vi "AddCustomError.vi"(1 "error in (no error)":errorcluster, 2 "source":string, 3 "code":i32, 4 "Error?":bool) -> (0 "error in (no error) 2":errorcluster)   [LabVIEW 2013]
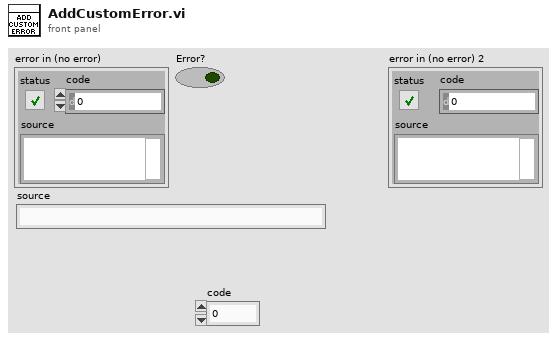
[diagram p1: front panel]
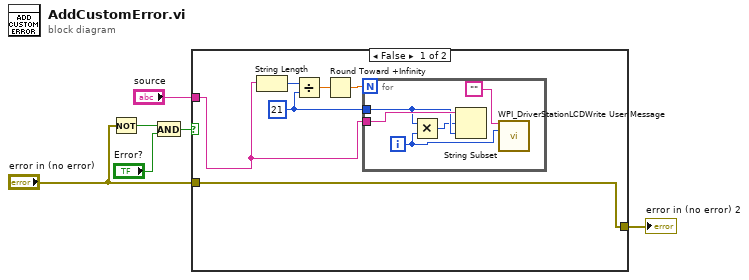
[diagram p0: block diagram]
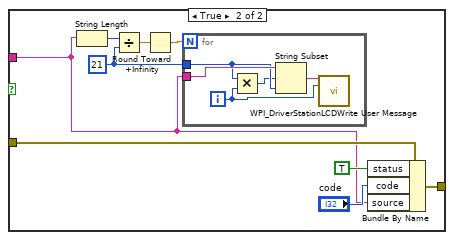
[diagram p2: hidden frame]
diagram:
  n1 = Not(x="error in (no error)") -> (.not. x?=w5:bool)
  n2 = And(x=w5, y="Error?") -> (x .and. y?=w6:bool)
  n3 = case shown="False" w6 {
    tunnel: "error in (no error)" -> [w12 w26]
    tunnel: [w12 w24] -> w2
    tunnel: "source" -> [w7 w18]
    frame False {
      w11 = 21 ("y")
      n4 = String Length(string=w7) -> (length=w8:i32)
      n5 = Divide(x=w8, y=w11) -> (x/y=w9:dbl)
      n6 = Round Toward +Infinity(x=w9) -> (ceil(x): smallest int >= x=w10:dbl)
      n7 = for {
        N: w10 -> [_]
        tunnel: w7 -> [w17]
        tunnel: w11 -> [w16]
        i -> [w15]
        n8 = Multiply(x=w16, y=w15) -> (x*y=w14:i32)
        n9 = String Subset(string=w17, offset (0)=w14, length (rest)=w16) -> ()  [unwired: 1 out]
        n10 = call <vilib>:"WPI_DriverStationLCDWrite User Message.vi"("line text"="", "line"=w15) -> ()  [unwired: 13 in, 1 out]
      }
    }
    frame True {
      w19 = 21 ("y")
      n11 = String Length(string=w18) -> (length=w22:i32)
      n12 = Divide(x=w22, y=w19) -> (x/y=w21:dbl)
      n13 = Round Toward +Infinity(x=w21) -> (ceil(x): smallest int >= x=w20:dbl)
      n14 = for {
        N: w20 -> [_]
        tunnel: w18 -> [w31]
        tunnel: w19 -> [w30]
        i -> [w29]
        n15 = Multiply(x=w30, y=w29) -> (x*y=w28:i32)
        n16 = String Subset(string=w31, offset (0)=w28, length (rest)=w30) -> (substring=w27:string)
        n17 = call <vilib>:"WPI_DriverStationLCDWrite User Message.vi"("line text"=w27, "line"=w29) -> ()  [unwired: 13 in, 1 out]
      }
      n18 = Bundle By Name(cluster=w26, "status"=TRUE, "code"="code", "source"=w18) -> (w24:errorcluster)
    }
  }
  "error in (no error) 2" <- w2
